vi "Monitor2DAQ.vi"(0 "instrument in":T2, 11 "error in":errorcluster, 13 "numSamples":i32=-1) -> (4 "instrument out":T2, 6 "wfm":waveform(dbl)[](array[waveform]), 15 "error out":errorcluster)   [LabVIEW 2013]
uses:
  <instrlib>/niScope/Acquire/Fetch/niScope Multi Fetch WDT.vi
panel:
  out "actualSamples 3":i32
  out "actualSamples 2":i32
  out "Chan 2 params":T1
  out "actualSamples 1":i32
  out "actualSamples 0":i32
  out "Chan 1 params":T1
  out "Chan 0 params":T1
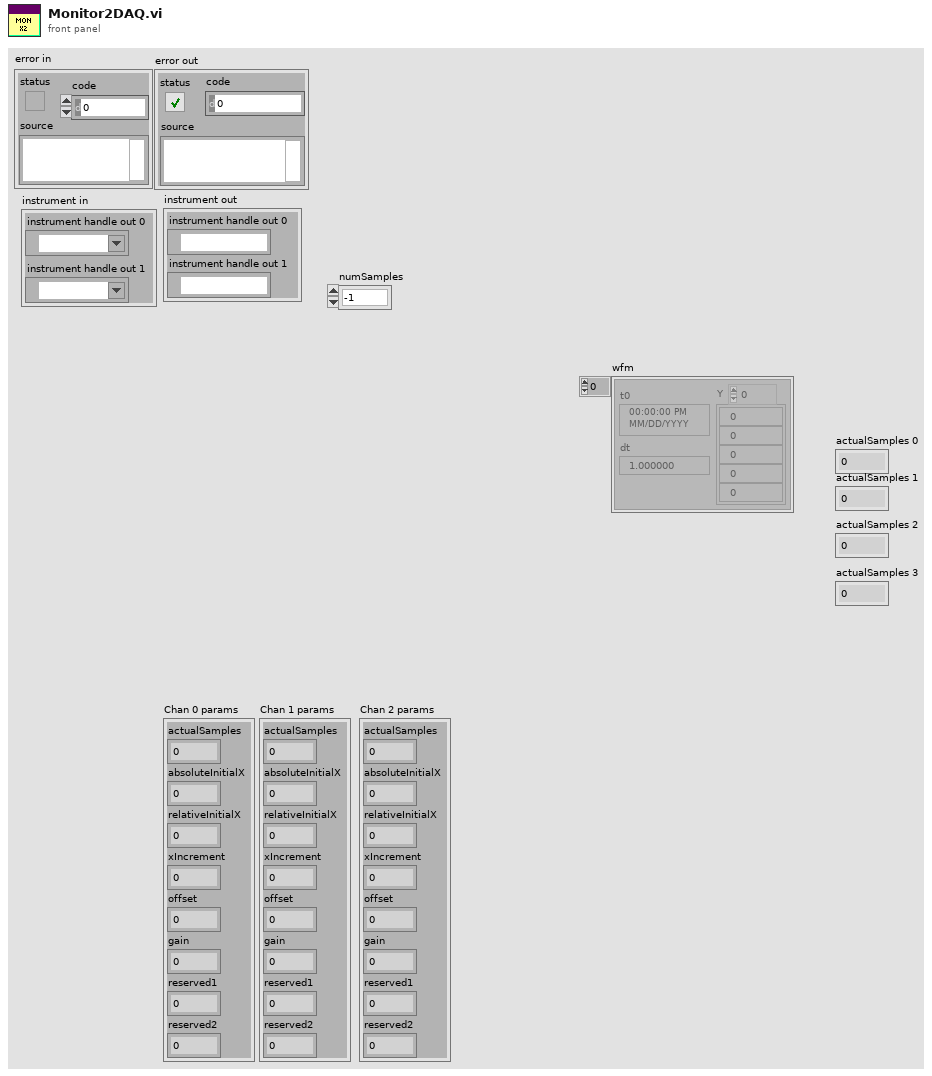
[diagram p1: front panel]
types:
  T1 = cluster{"actualSamples":i32, "absoluteInitialX":dbl, "relativeInitialX":dbl, "xIncrement":dbl, "offset":dbl, "gain":dbl, "reserved1":dbl, "reserved2":dbl}
  T2 = cluster{"instrument handle out 0":refnum<k15>, "instrument handle out 1":refnum<k15>}
  T3 = cluster{"actualSamples":i32, "absoluteInitialX":dbl, "relativeInitialX":dbl, "xIncrement":dbl, "offset":dbl, "gain":dbl, "reserved1":dbl, "reserved2":dbl}[]
  T4 = cluster{"instrument handle out":refnum<k15>, "instrument handle out":refnum<k15>}
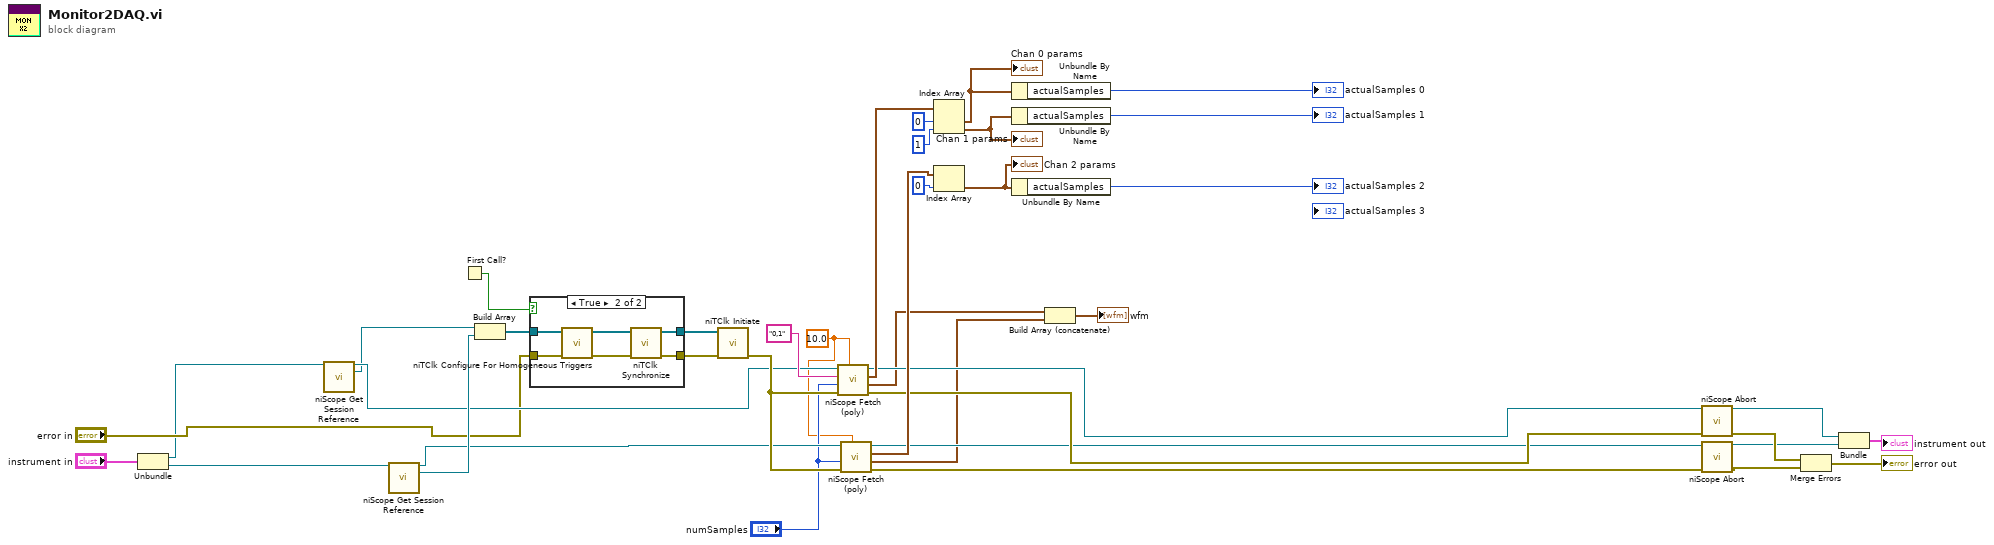
[diagram p0: block diagram]
diagram:
  w6 = 10.0 ("timeout")
  n1 = Unbundle("instrument in") -> ("instrument handle out 0"=w4:refnum<k15>, "instrument handle out 1"=w3:refnum<k15>)
  n2 = call <instrlib>:"niScope Get Session Reference.vi"("instrument handle"=w4) -> ("instrument handle out"=w16:refnum<k15>, "session reference"=w1:refnum<k20>)  [unwired: 12 in, 1 out]
  n3 = call <instrlib>:"niScope Get Session Reference.vi"("instrument handle"=w3) -> ("instrument handle out"=w15:refnum<k15>, "session reference"=w37:refnum<k20>)  [unwired: 12 in, 1 out]
  n4 = First Call?() -> (First Call?: T/F=w2:bool)
  n5 = Build Array(w1, w37) -> (w38:refnum<k20>[])
  n6 = case shown="True" w2 {
    tunnel: w38 -> [w42 w48]
    tunnel: [w41 w47] -> w26
    tunnel: [w42 w46] -> w25
    tunnel: "error in" -> [w41 w43]
    frame False {
    }
    frame True {
      n7 = call <instrlib>:"niTClk Configure For Homogeneous Triggers.vi"("error in (no error)"=w43, "sessions"=w48) -> ("error out"=w45:errorcluster, "sessions out"=w44:refnum<k20>[])  [unwired: 8 in]
      n8 = call <instrlib>:"niTClk Synchronize.vi"("error in (no error)"=w45, "sessions"=w44) -> ("error out"=w47:errorcluster, "sessions out"=w46:refnum<k20>[])  [unwired: 8 in]
    }
  }
  n9 = call <instrlib>:"niTClk Initiate.vi"("error in (no error)"=w26, "sessions"=w25) -> ("error out"=w24:errorcluster)  [unwired: 8 in, 1 out]
  n10 = call-poly <instrlib>:"niScope Fetch (poly).vi"("timeout"=w6, "error in"=w24, "numSamples"="numSamples", "channels"="0,1", "instrument handle"=w16) -> ("error out"=w20:errorcluster, "wfm"=w9:waveform(dbl)[], "wfm info"=w31:T3, "instrument handle out"=w19:refnum<k15>)  [unwired: 1 in, 2 out]
  n11 = call-poly <instrlib>:"niScope Fetch (poly).vi"("timeout"=w6, "error in"=w24, "numSamples"="numSamples", "instrument handle"=w15) -> ("error out"=w18:errorcluster, "wfm"=w8:waveform(dbl)[], "wfm info"=w21:T3, "instrument handle out"=w17:refnum<k15>)  [unwired: 2 in, 2 out]
  n12 = Index Array(array=w31, index #1=0 ("index"), index #2=1 ("index")) -> (element #1=w33:T1, element #2=w32:T1)
  "Chan 0 params" <- w33
  "Chan 1 params" <- w32
  n13 = Index Array(array=w21, index=0) -> (element=w22:T1)
  "Chan 2 params" <- w22
  n14 = Unbundle By Name(w33) -> ("actualSamples"=→"actualSamples 0":i32)
  n15 = Unbundle By Name(w32) -> ("actualSamples"=→"actualSamples 1":i32)
  n16 = Unbundle By Name(w22) -> ("actualSamples"=→"actualSamples 2":i32)
  n17 = Build Array (concatenate)(w9, w8) -> (→"wfm":waveform(dbl)[])
  n18 = call <instrlib>:"niScope Abort.vi"("instrument handle"=w19, "error in"=w20) -> ("instrument handle out"=w13:refnum<k15>, "error out"=w12:errorcluster)  [unwired: 12 in]
  n19 = call <instrlib>:"niScope Abort.vi"("instrument handle"=w17, "error in"=w18) -> ("instrument handle out"=w10:refnum<k15>, "error out"=w11:errorcluster)  [unwired: 12 in]
  n20 = Merge Errors(w12, w11) -> (→"error out":errorcluster)
  n21 = Bundle("instrument handle out"=w13, "instrument handle out"=w10) -> (→"instrument out":T4)  [unwired: 1 in]
